vi "Floor_Surface_Level.vi"(3 "Simulate/Run":T1, 4 "Traverse Setups":string[](array[string]), 5 "Position In":sgl[](array[numeric])=[0.0, 0.0, 0.0] format="%#.2f") -> (0 "Correct array":bool, 1 "Z Offset":sgl, 2 "Position Out":sgl[](array[numeric]) format="%#.2f")   [LabVIEW 2015]
uses:
  Controls/User_Specific_mode.ctl
  File/Setup_Filetype.ctl
  ADAM Client/Sub VIs/ADAM Controls/Update_scan_value.ctl
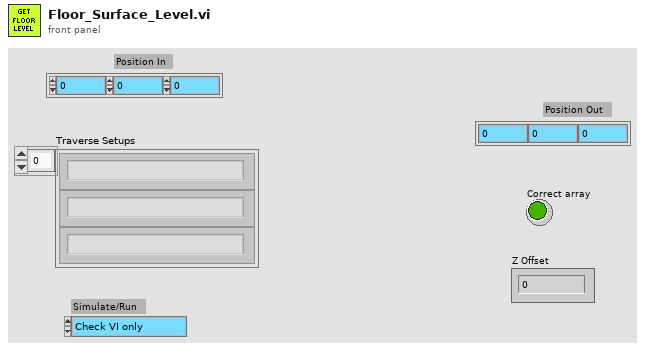
[diagram p1: front panel]
types:
  T1 = typedef "User_Specific_mode.ctl" = enum16{"Check VI only", "Run VI"}
  T2 = typedef "Setup_Filetype.ctl" = enum16{"Measurement Setups", "Calibration Setups", "General", "Results File Plotter Setups", "Speed Calib Tweaks"}
  T3 = typedef "Update_scan_value.ctl" = cluster{"Channel Name":string, "New Value":dbl}
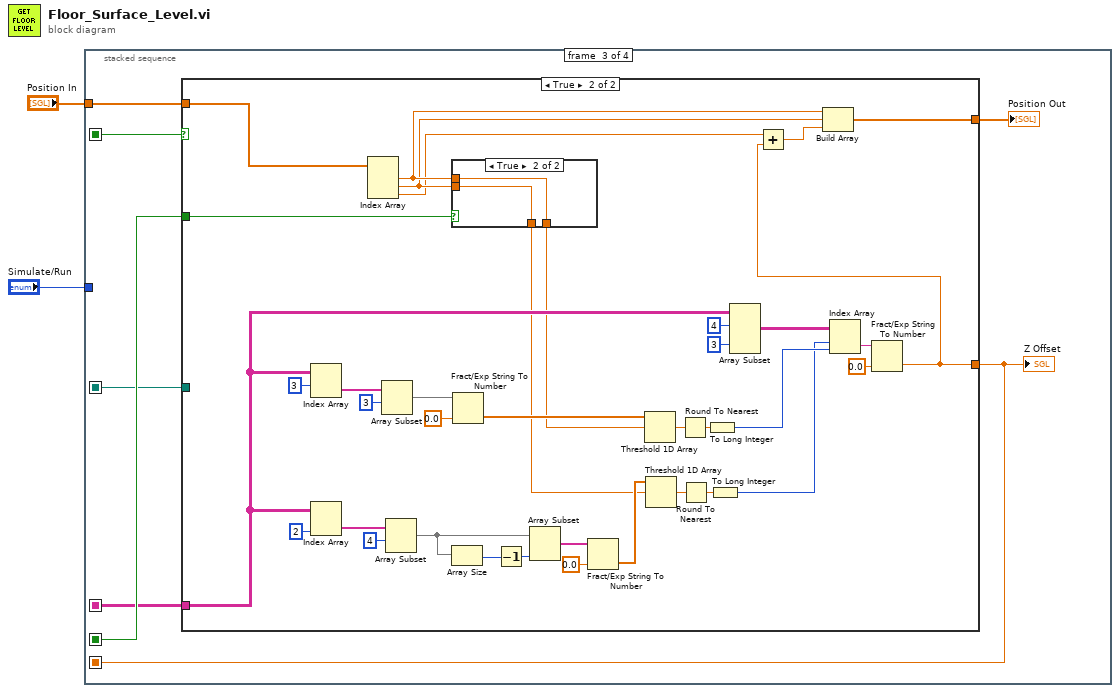
[diagram p0: block diagram]
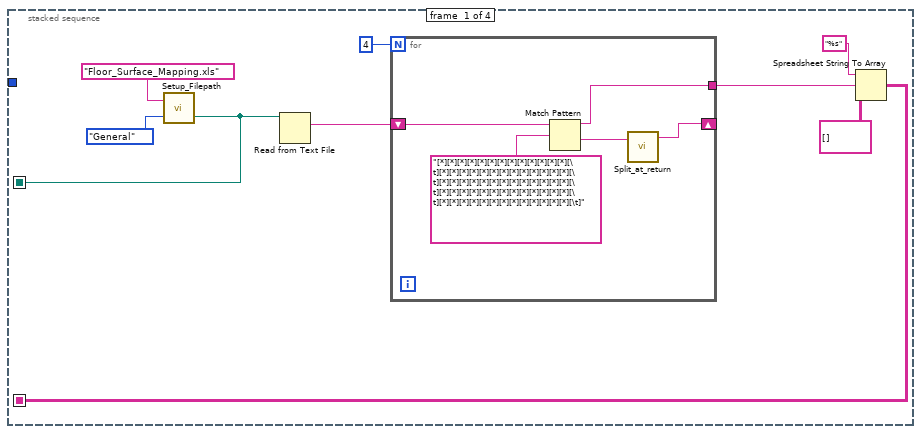
[diagram p2: hidden frame]
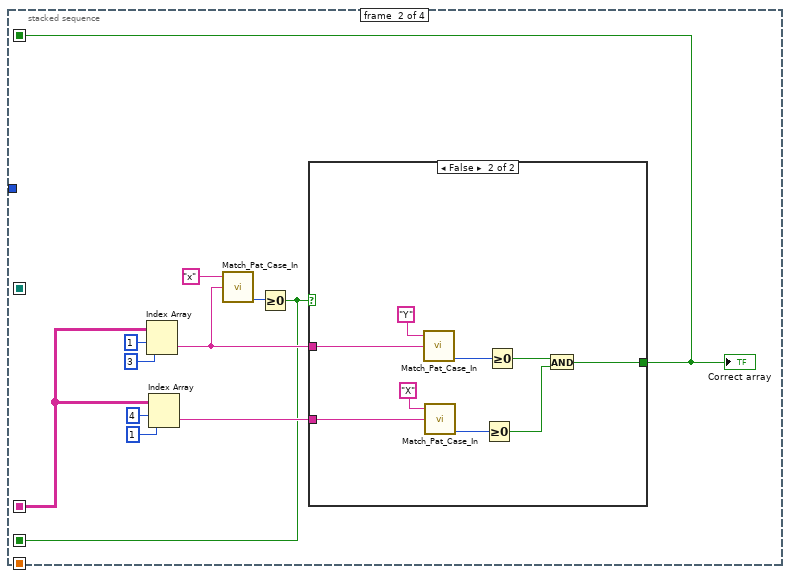
[diagram p3: hidden frame]
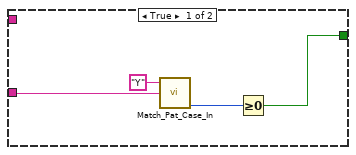
[diagram p4: hidden frame]
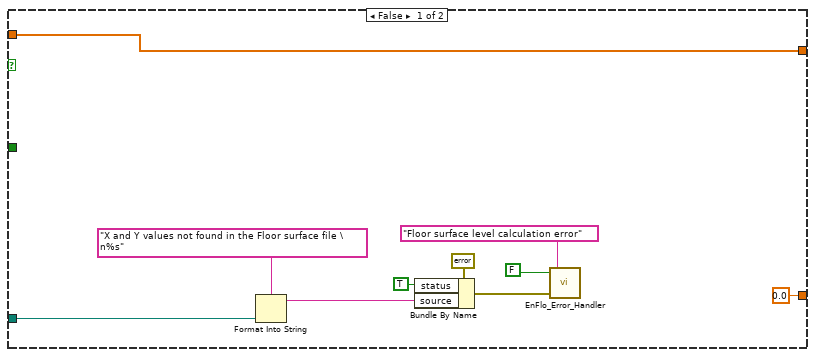
[diagram p5: hidden frame]
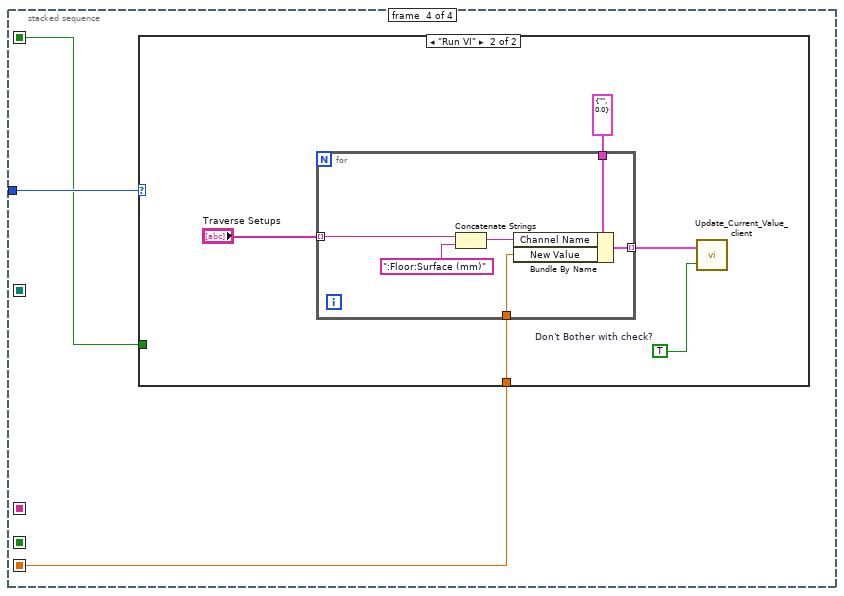
[diagram p7: hidden frame]
diagram:
  n1 = stacked-sequence {
    seq-local: [w6 _ _ _] -> [_ w22 w41 _]
    seq-local: [_ w18 _ _] -> [_ _ w47 _]
    seq-local: [_ _ w43 _] -> [_ _ _ w99]
    seq-local: [_ w17 _ _] -> [_ _ w44 w100]
    seq-local: [w3 _ _ _] -> [_ _ w42 _]
    tunnel: "Simulate/Run" -> [_ _ _ w101]
    tunnel: "Position In" -> [_ _ w45 _]
    frame #0 {
      n2 = call "Setup_Filepath.vi"("Setup File Type"=Setup_Filetype."General", "Filename in"="Floor_Surface_Mapping.xls") -> ("Filename Out"=w3:path)  [unwired: 1 out]
      n3 = Read from Text File(file (use dialog)=w3) -> (text=w11:string)  [unwired: 3 in, 3 out]
      n4 = for {
        N: 4 -> [_]
        shift-right: [w13] -> _
        shift-left: w11 -> [w14]
        tunnel: [w12] -> w8
        n5 = Match Pattern(string=w14, regular expression="[*][*][*][*][*][*][*][*][*][*][*][*][*][\t][*][*][*][*][*][*][*][*][*][*][*][*][*][\t][*][*][*][*][*][*][*][*][*][*][*][*][*][\t][*][*][*][*][*][*][*][*][*][*][*][*][*][\t][*][*][*][*][*][*][*][*][*][*][*][*][*][\t]" ("String")) -> (before substring=w12:string, after substring=w15:string)  [unwired: 3 out]
        n6 = call "Split_at_return.vi"("String"=w15) -> ("after substring"=w13:string)  [unwired: 1 in, 3 out]
      }
      n7 = Spreadsheet String To Array(format string="%s", spreadsheet string=w8, array type (2D Dbl)=string[][] []) -> (array=w6:string[][])  [unwired: 1 in]
    }
    frame #1 {
      n8 = Index Array(array=w22, index (row)=1, index (col)=3) -> (element=w20:string)
      n9 = Index Array(array=w22, index (row)=4, index (col)=1) -> (element=w21:string)
      n10 = call "Match_Pat_Case_In.vi"("String to match"="x", "String"=w20) -> ("offset past match"=w19:i32)  [unwired: 1 in, 3 out]
      n11 = Greater Or Equal To 0?(x=w19) -> (x >= 0?=w18:bool)
      n12 = case shown="False" w18 {
        tunnel: w21 -> [w30 w39]
        tunnel: w20 -> [_ w37]
        tunnel: [w28 w32] -> w17
        frame True {
          n13 = call "Match_Pat_Case_In.vi"("String to match"="Y", "String"=w30) -> ("offset past match"=w29:i32)  [unwired: 1 in, 3 out]
          n14 = Greater Or Equal To 0?(x=w29) -> (x >= 0?=w28:bool)
        }
        frame False {
          n15 = call "Match_Pat_Case_In.vi"("String to match"="Y", "String"=w37) -> ("offset past match"=w36:i32)  [unwired: 1 in, 3 out]
          n16 = call "Match_Pat_Case_In.vi"("String to match"="X", "String"=w39) -> ("offset past match"=w35:i32)  [unwired: 1 in, 3 out]
          n17 = Greater Or Equal To 0?(x=w35) -> (x >= 0?=w34:bool)
          n18 = Greater Or Equal To 0?(x=w36) -> (x >= 0?=w33:bool)
          n19 = And(x=w33, y=w34) -> (x .and. y?=w32:bool)
        }
      }
      "Correct array" <- w17
    }
    frame #2 {
      n20 = case shown="True" w44 {
        tunnel: w41 -> [_ w80]
        tunnel: w47 -> [_ w79]
        tunnel: [sgl 0.0 w74] -> w43
        tunnel: [w57 w71] -> w46
        tunnel: w45 -> [w57 w70]
        tunnel: w42 -> [w50 _]
        frame False {
          n21 = Format Into String(format string="X and Y values not found in the Floor surface file \n%s", w50) -> (resulting string=w48:string)  [unwired: 2 in, 1 out]
          n22 = Bundle By Name(cluster=errorcluster {"status"=FALSE, "code"=0, "source"=""} ("error in (no error)"), "status"=TRUE, "source"=w48) -> (w53:errorcluster)
          n23 = call "EnFlo_Error_Handler.vi"("error in (no error)"=w53, "Error Type"="Floor surface level calculation error", "Dialog Box (T)"=FALSE) -> ()  [unwired: 3 out]
        }
        frame True {
          n24 = Index Array(array=w80, index (row)=3) -> (element=w93:string[])  [unwired: 1 in]
          n25 = Index Array(array=w80, index (col)=2 ("index (row)")) -> (element=w89:string[])  [unwired: 1 in]
          n26 = Index Array(array=w70) -> (element #1=w76:sgl, element #2=w75:sgl, element #3=w73:sgl)  [unwired: 3 in]
          n27 = Array Subset(array=w93, index=3) -> (w86:string[])  [unwired: 1 in]
          n28 = Array Subset(array=w89, index=4) -> (w62:string[])  [unwired: 1 in]
          n29 = case shown="True" w79 {
            tunnel: w76 -> [w96 w98]
            tunnel: [w95 w98] -> w78
            tunnel: [w96 w97] -> w77
            tunnel: w75 -> [w95 w97]
            frame False {
            }
            frame True {
            }
          }
          n30 = Array Size(array=w62) -> (size(s)=w64:i32)
          n31 = Fract/Exp String To Number(string=w86, default (0 dbl)=sgl 0.0 ("default (0 DBL)")) -> (number=w85:sgl[])  [unwired: 2 in, 1 out]
          n32 = Decrement(x=w64) -> (x-1=w63:i32)
          n33 = Array Subset(array=w62, length=w63) -> (w61:string[])  [unwired: 1 in]
          n34 = Fract/Exp String To Number(string=w61, default (0 dbl)=sgl 0.0 ("default (0 DBL)")) -> (number=w82:sgl[])  [unwired: 2 in, 1 out]
          n35 = Threshold 1D Array(2:w78, 3:w85) -> (0:w84:sgl)  [unwired: 1 in]
          n36 = Threshold 1D Array(2:w77, 3:w82) -> (0:w83:sgl)  [unwired: 1 in]
          n37 = Round To Nearest(number=w84) -> (nearest integer value=w69:sgl)
          n38 = Round To Nearest(number=w83) -> (nearest integer value=w68:sgl)
          n39 = To Long Integer(number=w69) -> (32bit integer=w66:i32)
          n40 = To Long Integer(number=w68) -> (32bit integer=w65:i32)
          n41 = Array Subset(array=w80, index (row)=4 ("index"), index (col)=3 ("index")) -> (w67:string[][])  [unwired: 2 in]
          n42 = Index Array(array=w67, index (row)=w65, index (col)=w66) -> (element=w81:string)
          n43 = Fract/Exp String To Number(string=w81, default (0 dbl)=sgl 0.0 ("default (0 DBL)")) -> (number=w74:sgl)  [unwired: 2 in, 1 out]
          n44 = Add(x=w73, y=w74) -> (x+y=w72:sgl)
          n45 = Build Array(w76, w75, w72) -> (w71:sgl[])
        }
      }
      "Z Offset" <- w43
      "Position Out" <- w46
    }
    frame #3 {
      n46 = case shown="\"Run VI\"" w101 {
        tunnel: w100 -> [_ _]
        tunnel: w99 -> [_ w102]
        frame "Check VI only", Default {
        }
        frame "Run VI" {
          w103 = TRUE  # Don't Bother with check?
          n47 = for {
            tunnel: "Traverse Setups" -> [w111] mode=indexing
            tunnel: T3 {"Channel Name"="", "New Value"=0.0} ("Update Scan Value Cluster") -> [w110]
            tunnel: w102 -> [w109]
            tunnel: [w107] -> w104 mode=indexing
            n48 = Concatenate Strings(w111, ":Floor:Surface (mm)" ("string")) -> (w108:string)
            n49 = Bundle By Name(cluster=w110, "Channel Name"=w108, "New Value"=w109) -> (w107:T3)
          }
          n50 = call "Update_Current_Value_client.vi"("Don't Bother with check?"=w103, "Update array in"=w104) -> ()
        }
      }
    }
  }
